vi "AlliGator Add Plugins to Main Menu.vi"(8 "error in (no error)":errorcluster, 11 "Menu in":refnum<k9>) -> (0 "error out":errorcluster, 3 "Menu out":refnum<k9>)   [LabVIEW 2021, in "AlliGator Python Plugins.lvlib"]
doc: "Adds python functions to the corresponding AlliGator submenus.\n\nIf a submenu is empty, deactivates it."
uses:
  AlliGator Python Plugins.lvlib
  Menu/Menu.lvlib
  Time/Time.lvlib
panel:
  out "CPU (s)":dbl
  # "see the AlliGator License on the block diagram (Ctrl+E or Window:Show Block Diagram)"
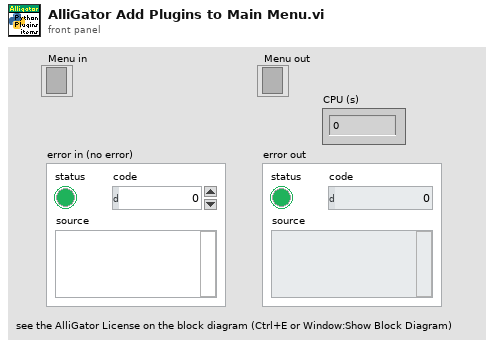
[diagram p1: front panel]
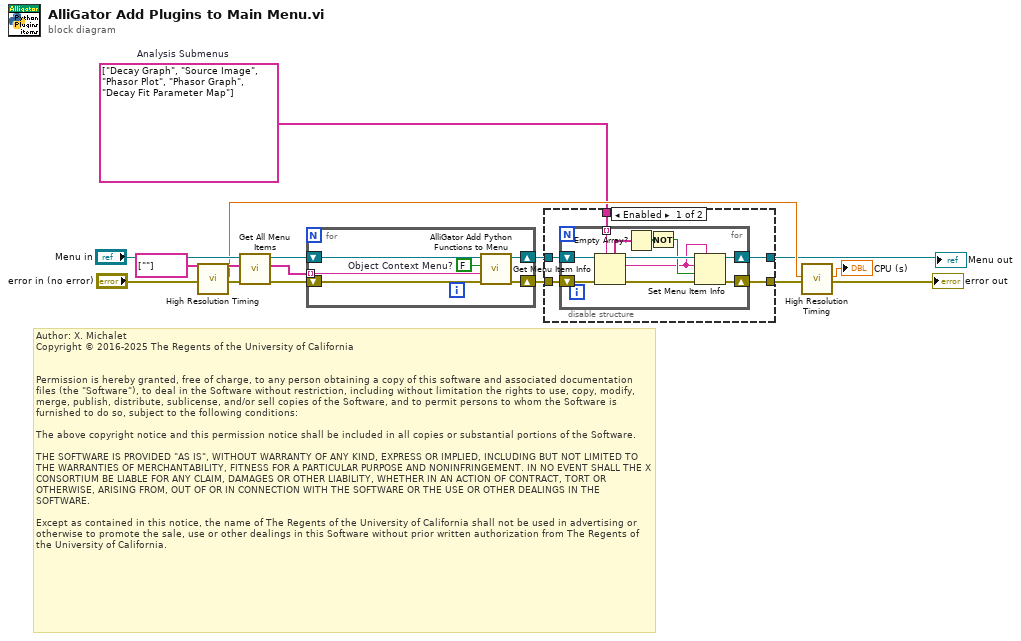
[diagram p0: block diagram]
diagram:
  w1 = string[] ["Decay Graph", "Source Image", "Phasor Plot", "Phasor Graph", "Decay Fit Parameter Map"]  # Analysis Submenus
  # "Author: X. Michalet\nCopyright © 2016-2025 The Regents of the University of California\n \n\nPermission is hereby granted, free of charge, to any person obtaining a copy of this software and associated documentation files (the \"Software\"), to deal in the Software without restriction, including without limitation the rights to use, copy, modify, merge, publish, distribute, sublicense, and/or sell copies of the Software, and to permit persons to whom the Software is furnished to do so, subject to the following conditions:\n\nThe above copyright notice and this permission notice shall be included in all copies or substantial portions of the Software.\n\nTHE SOFTWARE IS PROVIDED \"AS IS\", WITHOUT WARRANTY OF ANY KIND, EXPRESS OR IMPLIED, INCLUDING BUT NOT LIMITED TO THE WARRANTIES OF MERCHANTABILITY, FITNESS FOR A PARTICULAR PURPOSE AND NONINFRINGEMENT. IN NO EVENT SHALL THE X CONSORTIUM BE LIABLE FOR ANY CLAIM, DAMAGES OR OTHER LIABILITY, WHETHER IN AN ACTION OF CONTRACT, TORT OR OTHERWISE, ARISING FROM, OUT OF OR IN CONNECTION WITH THE SOFTWARE OR THE USE OR OTHER DEALINGS IN THE SOFTWARE.\n\nExcept as contained in this notice, the name of The Regents of the University of California shall not be used in advertising or otherwise to promote the sale, use or other dealings in this Software without prior written authorization from The Regents of the University of California."
  n1 = call "High Resolution Timing.vi"("Error In"="error in (no error)") -> ("elapsed (relative) seconds"=w8:dbl, "Error Out"=w10:errorcluster)  [unwired: 16 in, 1 out]
  n2 = call "Get All Menu Items.vi"("error in (no error)"=w10, "Item Tags (Default: All)"=string[] [""] ("Item Tags"), "Menu in"="Menu in") -> ("error out"=w12:errorcluster, "All Menu Tags"=w6:string[], "Menu out"=w14:refnum<k9>)  [unwired: 6 in]
  n3 = for {
    tunnel: w6 -> [w19] mode=indexing
    shift-right: [w18] -> w5
    shift-left: w14 -> [w21]
    shift-right: [w17] -> w4
    shift-left: w12 -> [w20]
    w16 = FALSE  # Object Context Menu?
    n4 = call "AlliGator Add Python Functions to Menu.vi"("error in (no error)"=w20, "Parent Menu Tag"=w19, "Object Context Menu?"=w16, "Menu in"=w21) -> ("error out"=w17:errorcluster, "Menu out"=w18:refnum<k9>)  [unwired: 6 in]
  }
  n5 = disable-structure shown="Enabled" {
    disable-tunnel: w5 -> [w26 w39]
    disable-tunnel: w4 -> [w25 w38]
    disable-tunnel: [w24 w38] -> w3
    disable-tunnel: [w23 w39] -> w2
    disable-tunnel: w1 -> [w22 _]
    frame Enabled {
      n6 = for {
        shift-right: [w28] -> w23
        shift-left: w26 -> [w37]
        shift-right: [w29] -> w24
        shift-left: w25 -> [w36]
        tunnel: w22 -> [w35] mode=indexing
        n7 = Get Menu Item Info(7:w35, 8:w36, 11:w37) -> (0:w32:errorcluster, 2:w27:string, 3:w33:refnum<k9>, 5:w34:string[])  [unwired: 3 out]
        n8 = Empty Array?(array=w34) -> (empty?=w31:bool)
        n9 = Not(x=w31) -> (.not. x?=w30:bool)
        n10 = Set Menu Item Info(7:w27, 8:w32, 9:w30, 10:w27, 11:w33) -> (0:w29:errorcluster, 3:w28:refnum<k9>)  [unwired: 2 in]
      }
    }
    frame Disabled {
    }
  }
  "Menu out" <- w2
  n11 = call "High Resolution Timing.vi"("relative seconds (NaN)"=w8, "Error In"=w3) -> ("elapsed (relative) seconds"=→"CPU (s)":dbl, "Error Out"=→"error out":errorcluster)  [unwired: 15 in, 1 out]
